vi "Init Bfr Tx - UDP Connection.vi"(8 "error in (no error)":errorcluster, 11 "Tx Loop Data in":T1={"General Resources"={"Packet Name"="", "Packet ID"=0, "Local IP Address"="", "Local Port"=0, "Multicast"=FALSE, "Multicast IP Address"=0, "Header Info"=[], "Byte Order"=enum."big-endian, network order", "Channel Data Types"=[], "Duplex Packets"=refnum}, "Header Details"={"Packet Size"=0, "Protocol Revision"=0, "System Definition Version"=0, "Source Node Name"="", "Packet ID"=0, "Number of Channels"=0, "Static Header Size"=0, "Total Header Size"=0, "CustomHeaderLogic"={"CustomHeaderON"=FALSE, "CustomHeaderLogic"=""}}, "Buffer Resources"={"Data Buffer"=0, "Pointer Encoding"=enum."Direct Encoding", "Buffer Size"=0, "Buffer Size (I32)"=0, "Raw Buffer Data"=[], "Is Buffered"=FALSE, "External Buffer"=FALSE, "Prepend Header"=FALSE, "Valid Buffer"=FALSE}, "Runtime Resources"={"Connection ID"=refnum, "Transmit Option"=enum."Always", "Destination IP Address"=0, "Destination Port"=0, "Multicast IP Address"=0, "TTL"=0, "Multicast"=FALSE, "Port as Channel"=FALSE, "ExecutionConfig"={"Loop Period"=0, "RT Loop Period"=-2, "Untimed Period"=0, "Target Processor"=0, "Priority"=0, "Thread Management"=enum."Untimed (Default)"}}, "Echo Resources"={"Transmit Echo Option"=enum."PCL Reset", "Packet Count"=0.0, "Counter Increment"=0.0, "Transmit Values"=[]}, "Buffer Option Support"={"Buffer Option"=enum."Static Buffer", "Sim Option"=enum."No Simulation"}, "Channel Resources"={"Transmit Flag"=refnum, "Transmit Echo"=refnum, "Transmit Bytes"=refnum, "Port Channel"=refnum, "Buffer (External)"=refnum, "Buffer (Local)"=refnum, "Timestamp"=refnum}, "Debug Resources"={"Debug Mode"=FALSE, "Debug Log File"=refnum, "Packet Name"=""}} {"Buffer Resources"."Data Buffer" format="%016x"}) -> (0 "error out":errorcluster, 3 "Tx Loop Data out":T1={"General Resources"={"Packet Name"="", "Packet ID"=0, "Local IP Address"="", "Local Port"=0, "Multicast"=FALSE, "Multicast IP Address"=0, "Header Info"=[], "Byte Order"=enum."big-endian, network order", "Channel Data Types"=[], "Duplex Packets"=refnum}, "Header Details"={"Packet Size"=0, "Protocol Revision"=0, "System Definition Version"=0, "Source Node Name"="", "Packet ID"=0, "Number of Channels"=0, "Static Header Size"=0, "Total Header Size"=0, "CustomHeaderLogic"={"CustomHeaderON"=FALSE, "CustomHeaderLogic"=""}}, "Buffer Resources"={"Data Buffer"=0, "Pointer Encoding"=enum."Direct Encoding", "Buffer Size"=0, "Buffer Size (I32)"=0, "Raw Buffer Data"=[], "Is Buffered"=FALSE, "External Buffer"=FALSE, "Prepend Header"=FALSE, "Valid Buffer"=FALSE}, "Runtime Resources"={"Connection ID"=refnum, "Transmit Option"=enum."Always", "Destination IP Address"=0, "Destination Port"=0, "Multicast IP Address"=0, "TTL"=0, "Multicast"=FALSE, "Port as Channel"=FALSE, "ExecutionConfig"={"Loop Period"=0, "RT Loop Period"=-2, "Untimed Period"=0, "Target Processor"=0, "Priority"=0, "Thread Management"=enum."Untimed (Default)"}}, "Echo Resources"={"Transmit Echo Option"=enum."PCL Reset", "Packet Count"=0.0, "Counter Increment"=0.0, "Transmit Values"=[]}, "Buffer Option Support"={"Buffer Option"=enum."Static Buffer", "Sim Option"=enum."No Simulation"}, "Channel Resources"={"Transmit Flag"=refnum, "Transmit Echo"=refnum, "Transmit Bytes"=refnum, "Port Channel"=refnum, "Buffer (External)"=refnum, "Buffer (Local)"=refnum, "Timestamp"=refnum}, "Debug Resources"={"Debug Mode"=FALSE, "Debug Log File"=refnum, "Packet Name"=""}} {"Buffer Resources"."Data Buffer" format="%016x"})   [LabVIEW 2019, in "UDP-Custom-Device Engine.lvlib"]
uses:
  UDP-Custom-Device Engine.lvlib
  Types/Engine - Buffered Tx Loop Data.ctl
  Types/Engine - General Resources.ctl
  <vilib>/NI VeriStand/VeriStand Data/Typedefs/Typedefs.Data Types.ctl
  Shared/Types/Shared - Duplex Settings.ctl
  Shared/Types/Shared - Header Details.ctl
  Shared/Types/Shared - Custom Header.ctl
  Types/Engine - Buffer Resources.ctl
  Shared/Types/Shared - Pointer Encoding.ctl
  Types/Engine - Tx Runtime Resources.ctl
  Shared/Types/Shared - Transmit Flag Options.ctl
  Types/Engine - Execution Config.ctl
  Shared/Types/Shared - Thread Management.ctl
  Types/Engine - Tx Echo Resources.ctl
  Shared/Types/Shared - Transmit Echo Options.ctl
  Types/Engine - Buffered Tx Buffer Option Support.ctl
  Shared/Types/Shared - Transmit Buffer Options.ctl
  Shared/Types/Shared - Transmit Sim Options.ctl
  Types/Engine - Buffered Tx Channel Refs.ctl
  <vilib>/NI/NIVS Inline Async API/_Data Access Engine/Data Access Engine/Types/Read.DVR.ctl
  <vilib>/NI/NIVS Inline Async API/_Data Access Engine/Access Type Classes/Read/Read.lvclass
  <vilib>/NI/NIVS Inline Async API/_Data Access Engine/Data Access Engine/Types/Write.DVR.ctl
  <vilib>/NI/NIVS Inline Async API/_Data Access Engine/Access Type Classes/Write/Write.lvclass
  Types/Engine - Debug Resources.ctl
  <vilib>/Utility/tcp.llb/UDP Multicast Write-Only Open.vi
  Shared/UDP-Custom-Device Shared.lvlib
  <vilib>/NI/NIVS Inline Async API/_Data Access Engine/Data Access Engine/Data Access Engine.lvclass
  <vilib>/NI VeriStand/VeriStand Data/VeriStand Data.lvlib
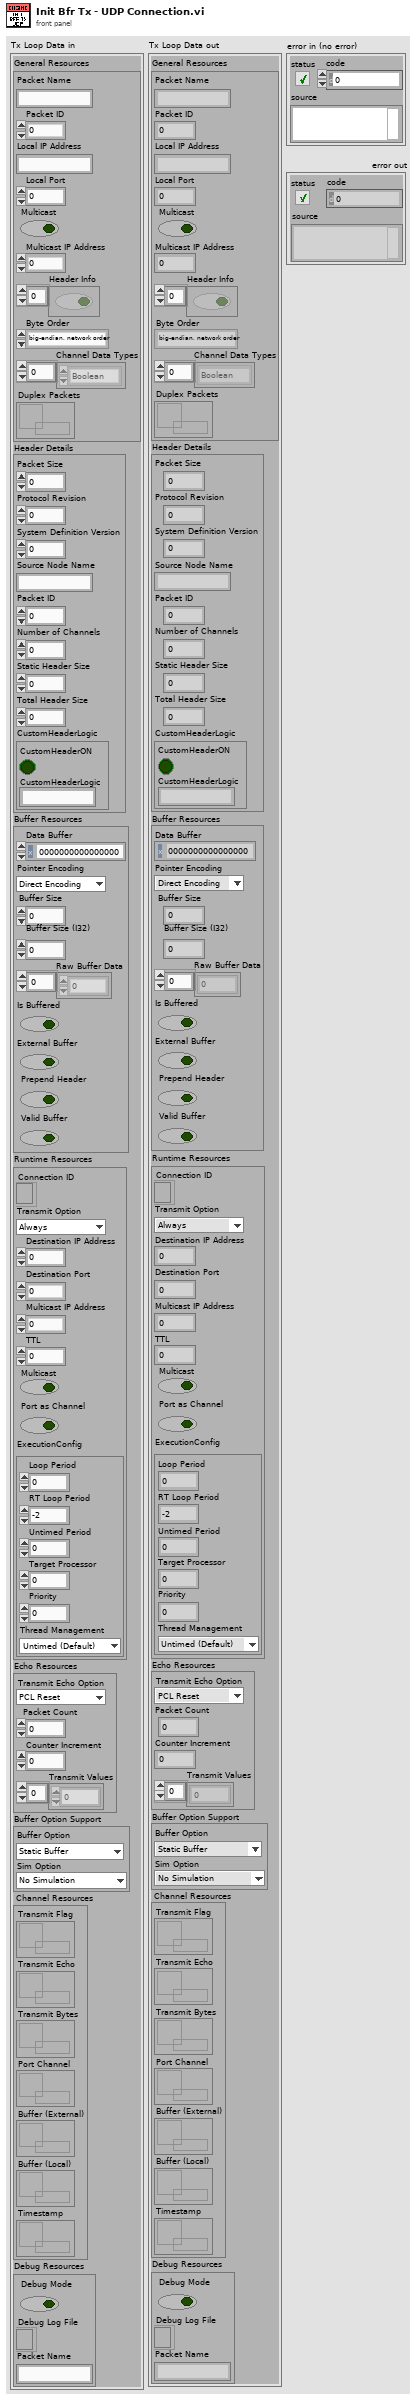
[diagram p1: front panel]
types:
  T1 = typedef "UDP-Custom-Device Engine.lvlib/Engine - Buffered Tx Loop Data.ctl" = cluster{"General Resources":T2, "Header Details":T4, "Buffer Resources":T6, "Runtime Resources":T8, "Echo Resources":T12, "Buffer Option Support":T14, "Channel Resources":T17, "Debug Resources":T20}
  T2 = typedef "UDP-Custom-Device Engine.lvlib/Engine - General Resources.ctl" = cluster{"Packet Name":string, "Packet ID":i32, "Local IP Address":string, "Local Port":i32, "Multicast":bool, "Multicast IP Address":u32, "Header Info":bool[], "Byte Order":enum16{"big-endian, network order", "native, host order", "little-endian"}, "Channel Data Types":T3[], "Duplex Packets":refnum<data-value>}
  T3 = typedef "VeriStand Data.lvlib/Typedefs.Data Types.ctl" = enum16{"Boolean", "Single", "Double", "I8", "I16", "I32", "I64", "U8", "U16", "U32", "U64"}
  T4 = typedef "UDP-Custom-Device Shared.lvlib/Shared - Header Details.ctl" = cluster{"Packet Size":u16, "Protocol Revision":u8, "System Definition Version":u64, "Source Node Name":string, "Packet ID":u32, "Number of Channels":u32, "Static Header Size":u16, "Total Header Size":u16, "CustomHeaderLogic":T5}
  T5 = typedef "UDP-Custom-Device Shared.lvlib/Shared - Custom Header.ctl" = cluster{"CustomHeaderON":bool, "CustomHeaderLogic":string}
  T6 = typedef "UDP-Custom-Device Engine.lvlib/Engine - Buffer Resources.ctl" = cluster{"Data Buffer":u64, "Pointer Encoding":T7, "Buffer Size":u64, "Buffer Size (I32)":i32, "Raw Buffer Data":u8[], "Is Buffered":bool, "External Buffer":bool, "Prepend Header":bool, "Valid Buffer":bool}
  T7 = typedef "UDP-Custom-Device Shared.lvlib/Shared - Pointer Encoding.ctl" = enum16{"Direct Encoding", "Conversion Encoding"}
  T8 = typedef "UDP-Custom-Device Engine.lvlib/Engine - Tx Runtime Resources.ctl" = cluster{"Connection ID":refnum<k16>, "Transmit Option":T9, "Destination IP Address":u32, "Destination Port":u16, "Multicast IP Address":u32, "TTL":u16, "Multicast":bool, "Port as Channel":bool, "ExecutionConfig":T10}
  T9 = typedef "UDP-Custom-Device Shared.lvlib/Shared - Transmit Flag Options.ctl" = enum16{"Always", "One-Shot", "Toggle"}
  T10 = typedef "UDP-Custom-Device Engine.lvlib/Engine - Execution Config.ctl" = cluster{"Loop Period":i64, "RT Loop Period":i64, "Untimed Period":u32, "Target Processor":i32, "Priority":i32, "Thread Management":T11}
  T11 = typedef "UDP-Custom-Device Shared.lvlib/Shared - Thread Management.ctl" = enum16{"Untimed (Default)", "Timed (High Priority)"}
  T12 = typedef "UDP-Custom-Device Engine.lvlib/Engine - Tx Echo Resources.ctl" = cluster{"Transmit Echo Option":T13, "Packet Count":dbl, "Counter Increment":dbl, "Transmit Values":dbl[]}
  T13 = typedef "UDP-Custom-Device Shared.lvlib/Shared - Transmit Echo Options.ctl" = enum16{"PCL Reset", "Counter", "Mirror"}
  T14 = typedef "UDP-Custom-Device Engine.lvlib/Engine - Buffered Tx Buffer Option Support.ctl" = cluster{"Buffer Option":T15, "Sim Option":T16}
  T15 = typedef "UDP-Custom-Device Shared.lvlib/Shared - Transmit Buffer Options.ctl" = enum16{"Static Buffer", "FIFO Buffer", "FIFO Buffer + Port"}
  T16 = typedef "UDP-Custom-Device Shared.lvlib/Shared - Transmit Sim Options.ctl" = enum16{"No Simulation", "Counter", "Full Buffer", "FIFO Test", "FIFO + Port Test"}
  T17 = typedef "UDP-Custom-Device Engine.lvlib/Engine - Buffered Tx Channel Refs.ctl" = cluster{"Transmit Flag":T18, "Transmit Echo":T19, "Transmit Bytes":T18, "Port Channel":T18, "Buffer (External)":T18, "Buffer (Local)":T19, "Timestamp":T18}
  T18 = typedef "Data Access Engine.lvlib/Data Access Engine.lvclass/Read.DVR.ctl" = refnum<data-value>
  T19 = typedef "Data Access Engine.lvlib/Data Access Engine.lvclass/Write.DVR.ctl" = refnum<data-value>
  T20 = typedef "UDP-Custom-Device Engine.lvlib/Engine - Debug Resources.ctl" = cluster{"Debug Mode":bool, "Debug Log File":refnum<file>, "Packet Name":string}
  T21 = typedef "UDP-Custom-Device Shared.lvlib/Shared - Duplex Settings.ctl" = cluster{"Transmit Packet ID":i32, "Receive Packet ID":i32, "Multicast":bool, "Multicast Address":string, "IP Address":string, "Port":u16, "TTL":u16, "Duplex Connection":refnum<k16>}
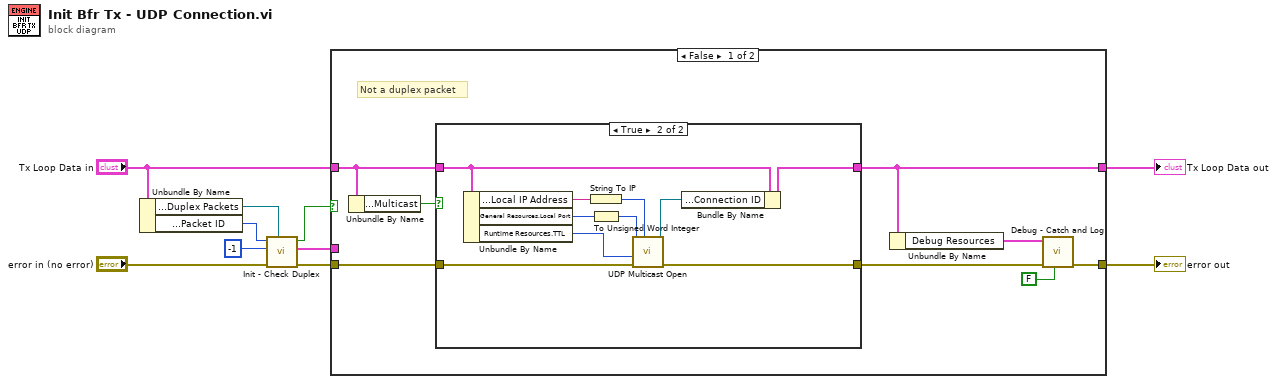
[diagram p0: block diagram]
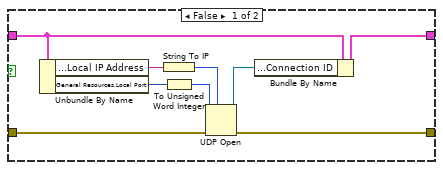
[diagram p2: hidden frame]
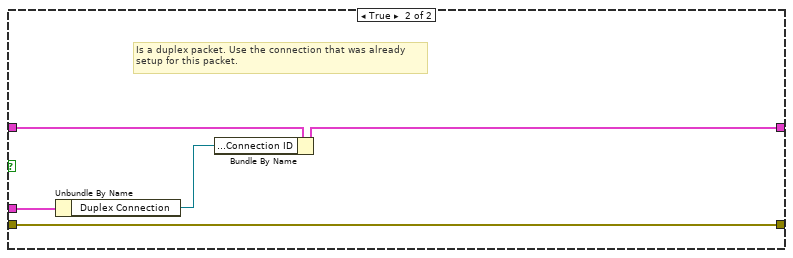
[diagram p3: hidden frame]
diagram:
  n1 = Unbundle By Name("Tx Loop Data in") -> ("General Resources.Duplex Packets"=w8:refnum<data-value>, "General Resources.Packet ID"=w5:i32)
  n2 = call "Init - Check Duplex.vi"("Duplex Packets"=w8, "error in (no error)"="error in (no error)", "Receive Packet ID"=-1, "Transmit Packet ID"=w5) -> ("error out"=w3:errorcluster, "Duplex Settings"=w2:T21, "Is Duplex?"=w6:bool)  [unwired: 5 in]
  n3 = case shown="False" w6 {
    tunnel: w3 -> [w18 w38]
    tunnel: [w13 w38] -> w10
    tunnel: [w11 w40] -> w9
    tunnel: "Tx Loop Data in" -> [w17 w41]
    tunnel: w2 -> [_ w39]
    frame False {
      # "Not a duplex packet"
      n4 = Unbundle By Name(w17) -> ("Runtime Resources.Multicast"=w16:bool)
      n5 = case shown="True" w16 {
        tunnel: w18 -> [w22 w32]
        tunnel: [w21 w31] -> w12
        tunnel: w17 -> [w20 w30]
        tunnel: [w19 w29] -> w11
        frame False {
          n6 = Unbundle By Name(w20) -> ("General Resources.Local IP Address"=w24:string, "General Resources.Local Port"=w27:i32)
          n7 = String To IP(1:w24) -> (0:w23:u32)
          n8 = To Unsigned Word Integer(number=w27) -> (unsigned 16bit integer=w25:u16)
          n9 = UDP Open(7:w23, 8:w22, 11:w25) -> (port=w26:refnum<k16>, 0:w21:errorcluster)  [unwired: 2 in, 1 out]
          n10 = Bundle By Name(cluster=w20, "Runtime Resources.Connection ID"=w26) -> (w19:T1)
        }
        frame True {
          n11 = Unbundle By Name(w30) -> ("General Resources.Local IP Address"=w34:string, "General Resources.Local Port"=w37:i32, "Runtime Resources.TTL"=w28:u16)
          n12 = String To IP(1:w34) -> (0:w33:u32)
          n13 = To Unsigned Word Integer(number=w37) -> (unsigned 16bit integer=w35:u16)
          n14 = call-poly <vilib>:"UDP Multicast Open.vi"("net address"=w33, "error in (no error)"=w32, "time-to-live (1)"=w28, "port"=w35) -> ("error out"=w31:errorcluster, "connection ID"=w36:refnum<k16>)  [unwired: 6 in]
          n15 = Bundle By Name(cluster=w30, "Runtime Resources.Connection ID"=w36) -> (w29:T1)
        }
      }
      n16 = Unbundle By Name(w11) -> ("Debug Resources"=w14:T20)
      n17 = call "Debug - Catch and Log.vi"("Clear Error?"=FALSE, "error in (no error)"=w12, "Debug Resources"=w14) -> ("error out"=w13:errorcluster)  [unwired: 8 in]
    }
    frame True {
      # "Is a duplex packet. Use the connection that was already\nsetup for this packet."
      n18 = Unbundle By Name(w39) -> ("Duplex Connection"=w42:refnum<k16>)
      n19 = Bundle By Name(cluster=w41, "Runtime Resources.Connection ID"=w42) -> (w40:T1)
    }
  }
  "Tx Loop Data out" <- w9
  "error out" <- w10
